vi "Gain Ranging FSM.vi"(0 "gain ranging.start sequence":bool, 5 "gain ranging.dwell time (cycles)":u32=4800, 7 "gain ranging.gain setting list":T5, 9 "gain ranging.manual request":T3) -> (4 "gain ranging.gain setting":fxp<+/-,16,12>, 6 "gain ranging.TX1/RX1 Port Value":T1=enum."TX1/RX2", 8 "gain ranging.start of sequence":bool, 10 "gain ranging.gain setting valid":bool)   [LabVIEW 2018]
uses:
  Host/SubVIs/TypeDefs/Gain Setting.ctl
  <instrlib>/niMmWave/ni3620/Config/v1/FPGA/Public/Typedefs/TX1 RX1 Port.ctl
  <vilib>/rvi/DataTransferAndStorage/Container/Common/niFpgaContainerGetUniqueNameForEmu.vi
  <vilib>/rvi/DataTransferAndStorage/Container/Common/niFpgaContainerSetEmuInfo.vi
  <vilib>/rvi/eio/common/nirviEmuReportErrorAndStop.vi
  <vilib>/rvi/DataTransferAndStorage/Container/Common/niFpgaContainerExecOnDevCompGetState.vi
  <vilib>/rvi/Emulation/niFpgaEmulationIsFPGAContextNoSignature.vi
  <vilib>/rvi/Emulation/niFpgaProcessEmulError.vi
  <vilib>/rvi/Emulation/niFpgaSctlEmulationGetInTimedLoop.vi
  <vilib>/rvi/errors/nirviReportUnexpectedCaseInternalError (U32).vi
  <vilib>/rvi/Memory/Memory_Emulation/niFpgaMemoryEmulationCacheClearOnFirstRun.vi
  <vilib>/rvi/Memory/Memory_Emulation/nirvimemoryEmulationManagerCache_MakeExclusive.vi
  <vilib>/rvi/Memory/Memory_Emulation/niFpgaMemoryEmulationValidateCache.vi
  <vilib>/rvi/Memory/Memory_Emulation/nirvimemoryEmulationManagerCache_InsertValue.vi
  <vilib>/Utility/error.llb/Clear Errors.vi
  <vilib>/rvi/Memory/Memory_Emulation/nirvimemoryEmulationManagerCache_ReleaseExclusive.vi
  <vilib>/rvi/Memory/Memory_Emulation/nirvimemoryEmulationManagerCache_GetValue.vi
  <vilib>/rvi/Memory/Memory_Emulation/nirvimemoryEmulationManagerCache_SetValue.vi
  <vilib>/rvi/Emulation/niFpgaSctlEmulationResourceMgr.vi
  <instrlib>/_niInstr/Basic Elements/v1/FPGA/Private/Count Up U16.vi
  <instrlib>/_niInstr/Basic Elements/v1/FPGA/Private/Count Down U32.vi
  <vilib>/rvi/LocalResourceManager/LocalResourceManager.xnode
  <vilib>/rvi/DataTransferAndStorage/Container/XNode/niFpgaContainer.xnode
  <vilib>/rvi/Memory/Memory_Emulation/niFpgaMemoryEmulationRefIn.vi
  <instrlib>/_niInstr/Basic Elements/v1/FPGA/niInstr Basic Elements v1 FPGA.lvlib
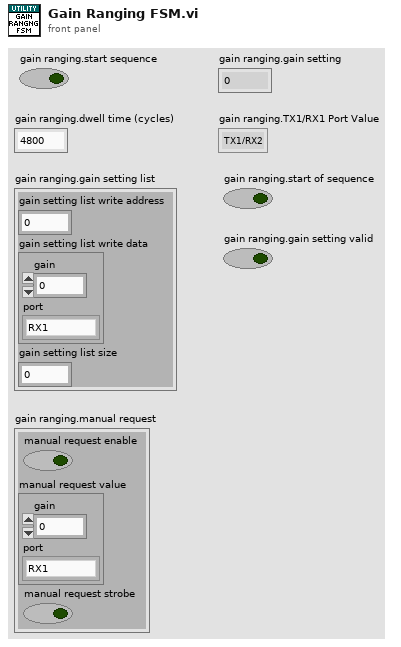
[diagram p1: front panel]
types:
  T1 = typedef "TX1 RX1 Port.ctl" = enum8{"RX1", "TX1/RX2"}
  T2 = typedef "Gain Setting.ctl" = cluster{"gain":fxp<+/-,16,12>, "port":T1}
  T3 = cluster{"manual request enable":bool, "manual request value":T2, "manual request strobe":bool}
  T4 = typedef "gain setting.ctl" = cluster{"gain":fxp<+/-,16,12>, "port":T1}
  T5 = cluster{"gain setting list write address":u32, "gain setting list write data":T4, "gain setting list size":u16}
  T6 = cluster{"gain":fxp<+/-,16,12>, "port":enum8{"RX1", "TX1/RX2"}}
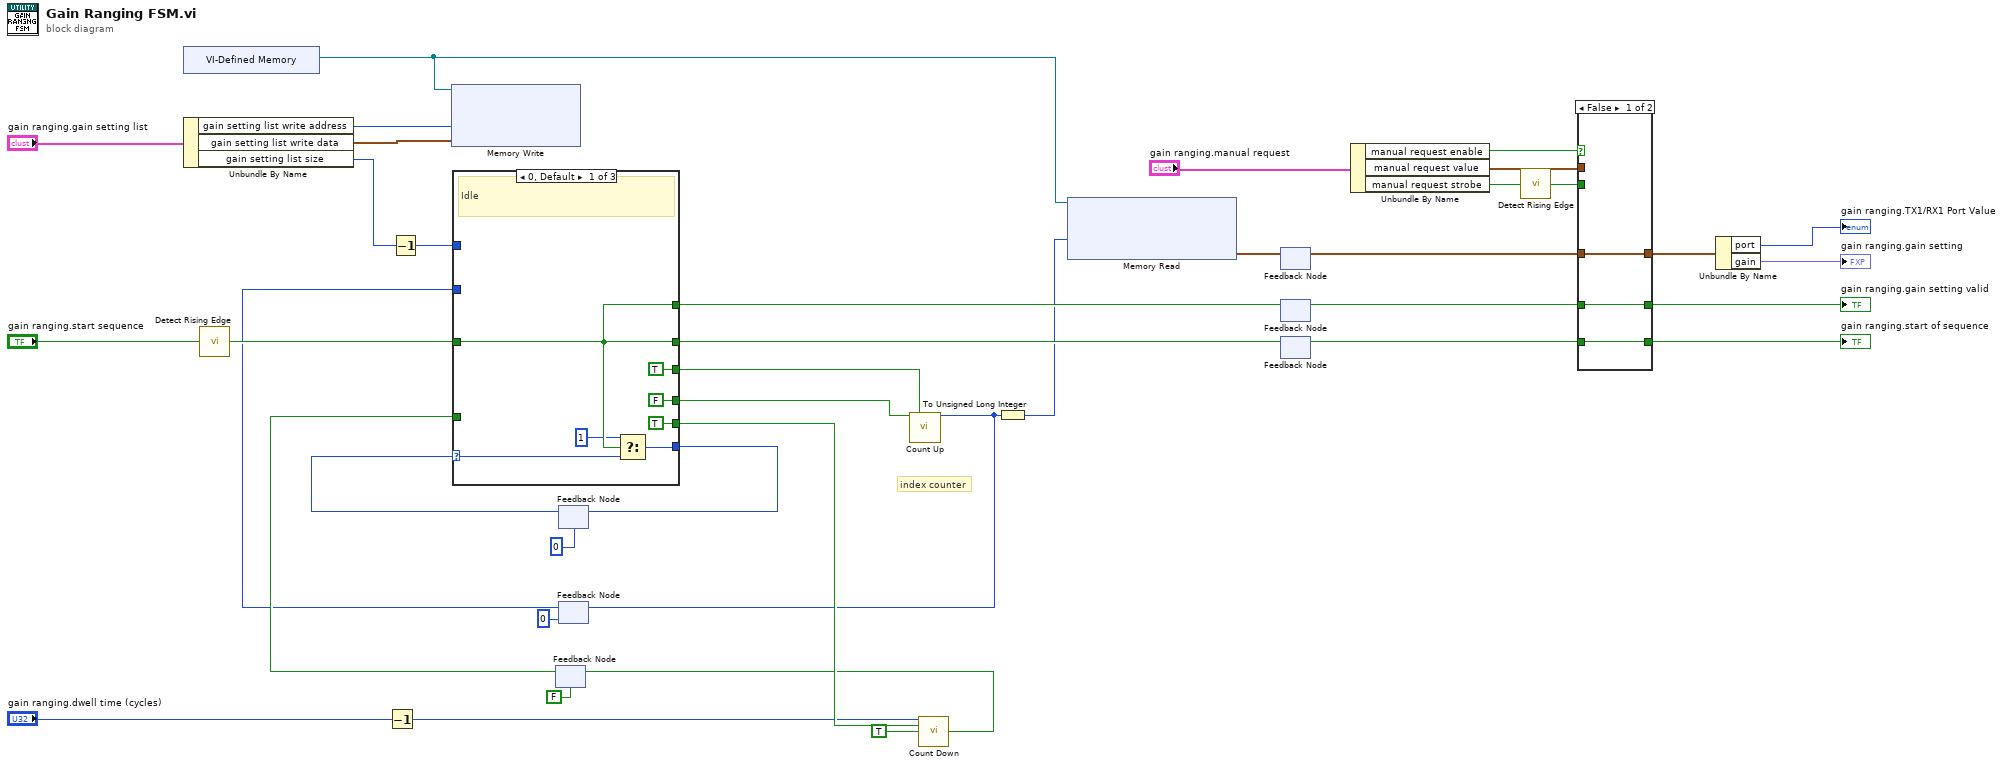
[diagram p0: block diagram]
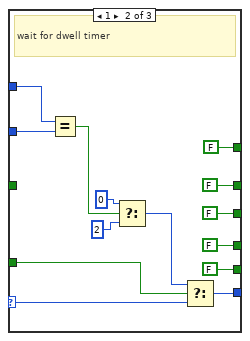
[diagram p2: hidden frame]
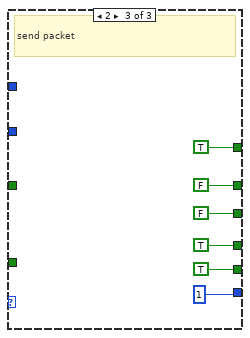
[diagram p3: hidden frame]
diagram:
  # "index counter"
  n1 = xnode "VI-Defined Memory"() -> ("Memory Out"=w14:refnum<k21>)
  n2 = Unbundle By Name("gain ranging.gain setting list") -> ("gain setting list write address"=w10:u32, "gain setting list write data"=w9:T4, "gain setting list size"=w8:u16)
  n3 = call <instrlib>:"Detect Rising Edge.vi"("signal"="gain ranging.start sequence") -> ("edge detected"=w29:bool)  [unwired: 14 in]
  n4 = Decrement(x="gain ranging.dwell time (cycles)") -> (x-1=w15:u32)
  n5 = Decrement(x=w8) -> (x-1=w18:u16)
  n6 = xnode "Memory Write"("Address"=w10, "Data"=w9, "Memory In"=w14) -> ()  [unwired: 1 out]
  n7 = feedback #1(FALSE ("terminal count")) -> (w22:bool)
  n8 = feedback #2(u8 0) -> (w30:u8)
  n9 = feedback #3(u16 0) -> (w19:u16)
  n10 = case shown="0, Default" w30 {
    selector: w30 -> [w47 w59 _]
    tunnel: w29 -> [w44 _ _]
    tunnel: [w46 w60 u8 1 ("t")] -> w28
    tunnel: [w44 FALSE FALSE] -> w39
    tunnel: [TRUE ("edge detected") FALSE ("edge detected") TRUE ("edge detected")] -> w27
    tunnel: [TRUE ("edge detected") FALSE ("edge detected") FALSE ("edge detected")] -> w25
    tunnel: [FALSE ("edge detected") FALSE ("edge detected") TRUE ("edge detected")] -> w24
    tunnel: w22 -> [_ w58 _]
    tunnel: w19 -> [_ w51 _]
    tunnel: w18 -> [_ w52 _]
    tunnel: [w44 FALSE ("edge detected") TRUE ("edge detected")] -> w37
    frame 0, Default {
      # "Idle"
      n11 = Select(t=u8 1, s=w44, f=w47) -> (s? t:f=w46:u8)
    }
    frame 1 {
      # "wait for dwell timer"
      n12 = Equal?(x=w52, y=w51) -> (x = y?=w49:bool)
      n13 = Select(t=u8 0, s=w49, f=u8 2 ("t")) -> (s? t:f=w50:u8)
      n14 = Select(t=w50, s=w58, f=w59) -> (s? t:f=w60:u8)
    }
    frame 2 {
      # "send packet"
    }
  }
  n15 = feedback-in #2(w28) -> ()
  n16 = call-poly <instrlib>:"Count Up.vi"("increment"=w24, "reset"=w25) -> ("count out"=w17:u16)  [unwired: 13 in]
  n17 = feedback-in #3(w17) -> ()
  n18 = call-poly <instrlib>:"Count Down.vi"("count in"=w15, "load"=w27, "decrement"=TRUE) -> ("terminal count"=w23:bool)  [unwired: 11 in, 1 out]
  n19 = feedback-in #1(w23) -> ()
  n20 = To Unsigned Long Integer(number=w17) -> (unsigned 32bit integer=w13:u32)
  n21 = xnode "Memory Read"("Address"=w13, "Memory In"=w14) -> ("Data"=w12:T6)  [unwired: 1 out]
  n22 = feedback #4() -> (w36:T6)  [unwired: 1 in]
  n23 = feedback-in #4(w12) -> ()
  n24 = feedback #5() -> (w38:bool)  [unwired: 1 in]
  n25 = feedback-in #5(w37) -> ()
  n26 = feedback #6() -> (w40:bool)  [unwired: 1 in]
  n27 = feedback-in #6(w39) -> ()
  n28 = Unbundle By Name("gain ranging.manual request") -> ("manual request enable"=w6:bool, "manual request value"=w5:T2, "manual request strobe"=w4:bool)
  n29 = call <instrlib>:"Detect Rising Edge.vi"("signal"=w4) -> ("edge detected"=w32:bool)  [unwired: 14 in]
  n30 = case shown="False" w6 {
    tunnel: [w70 w72] -> w3
    tunnel: w36 -> [w70 _]
    tunnel: [w68 w71] -> w35
    tunnel: w5 -> [_ w72]
    tunnel: w32 -> [_ w71]
    tunnel: w40 -> [w69 _]
    tunnel: [w69 w71] -> w34
    tunnel: w38 -> [w68 _]
    frame False {
    }
    frame True {
    }
  }
  "gain ranging.gain setting valid" <- w35
  "gain ranging.start of sequence" <- w34
  n31 = Unbundle By Name(w3) -> ("port"=→"gain ranging.TX1/RX1 Port Value":T1, "gain"=→"gain ranging.gain setting":fxp<+/-,16,12>)
